vi "B.4.путь каталога отчета.vi"() -> (3 "path_out":string)   [LabVIEW 2011]
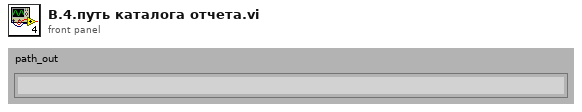
[diagram p1: front panel]
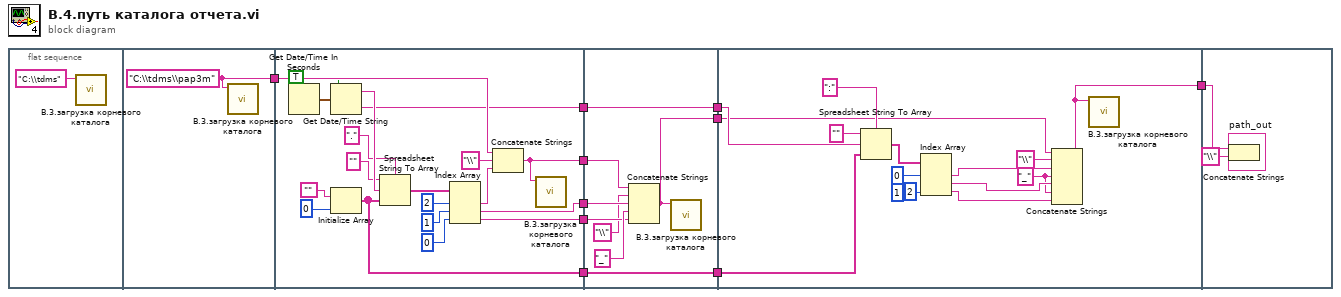
[diagram p0: block diagram]
diagram:
  n1 = flat-sequence {
    tunnel: [w12] -> w10
    tunnel: w10 -> [w23]
    tunnel: [w18] -> w9
    tunnel: [w17] -> w8
    tunnel: [w16] -> w7
    tunnel: [w15] -> w5
    tunnel: [w14] -> w3
    tunnel: w9 -> [w39]
    tunnel: w8 -> [w37]
    tunnel: w7 -> [w35]
    tunnel: [w34] -> w6
    tunnel: w5 -> [w34]
    tunnel: [w33] -> w4
    tunnel: w3 -> [w33]
    tunnel: [w32] -> w2
    tunnel: w6 -> [w53]
    tunnel: w4 -> [w54]
    tunnel: w2 -> [w41]
    tunnel: [w40] -> w1
    tunnel: w1 -> [w57]
    frame #0 {
      n2 = call "B.3.загрузка корневого каталога.vi"("path"="C:\\tdms") -> ()  [unwired: 10 in, 1 out]
    }
    frame #1 {
      w12 = "C:\\tdms\\pap3m" ("path")
      n3 = call "B.3.загрузка корневого каталога.vi"("path"=w12) -> ()  [unwired: 10 in, 1 out]
    }
    frame #2 {
      n4 = Get Date/Time In Seconds() -> (seconds since 1Jan1904=w31:timestamp)
      n5 = Get Date/Time String(seconds (now)=w31, want seconds? (F)=TRUE) -> (date string=w30:string, time string=w15:string)  [unwired: 1 in]
      n6 = Initialize Array("", 0 ("dimension size")) -> (w14:string[])
      n7 = Spreadsheet String To Array(delimiter (Tab)=".", format string="", spreadsheet string=w30, array type (2D Dbl)=w14) -> (array=w27:string[])
      n8 = Index Array(array=w27, index #1=2 ("index"), index #2=1 ("index"), index #3=0 ("index")) -> (element #1=w21:string, element #2=w18:string, element #3=w17:string)
      n9 = Concatenate Strings(w23, "\\" ("string"), w21) -> (w16:string)
      n10 = call "B.3.загрузка корневого каталога.vi"("path"=w16) -> ()  [unwired: 10 in, 1 out]
    }
    frame #3 {
      n11 = Concatenate Strings(w35, "\\" ("string"), w39, "_" ("string"), w37) -> (w32:string)
      n12 = call "B.3.загрузка корневого каталога.vi"("path"=w32) -> ()  [unwired: 10 in, 1 out]
    }
    frame #4 {
      w47 = "_" ("string")
      n13 = Spreadsheet String To Array(delimiter (Tab)=":", format string="", spreadsheet string=w53, array type (2D Dbl)=w54) -> (array=w50:string[])
      n14 = Index Array(array=w50, index #1=0 ("index"), index #2=1 ("index"), index #3=2 ("index")) -> (element #1=w49:string, element #2=w48:string, element #3=w46:string)
      n15 = Concatenate Strings(w41, "\\" ("string"), w49, w47, w48, w47, w46) -> (w40:string)
      n16 = call "B.3.загрузка корневого каталога.vi"("path"=w40) -> ()  [unwired: 10 in, 1 out]
    }
    frame #5 {
      n17 = Concatenate Strings(w57, "\\" ("string")) -> (→"path_out":string)
    }
  }
